vi "Robot_s Third Move.vi"(0 "Machine In":refnum<visa-resource-name>, 5 "Image Value From First Turn":dbl, 7 "Image  value From Second Turn":dbl, 9 "Index From First Move":i32, 11 "Index From Second Move":i32, 12 "error in":errorcluster) -> (4 "Machine Out":refnum<visa-resource-name>, 8 "Next Move":enum16{"Child's Turn", "Robot's Turn"}(ring), 15 "error out":errorcluster)   [LabVIEW 2018]
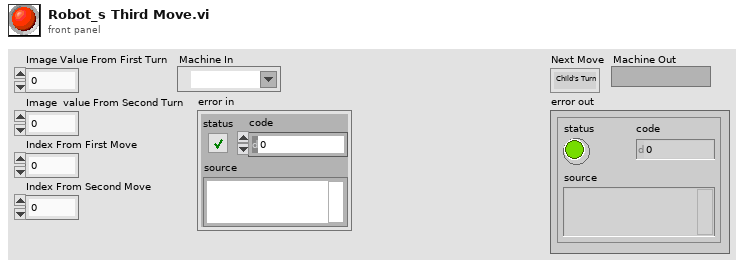
[diagram p1: front panel]
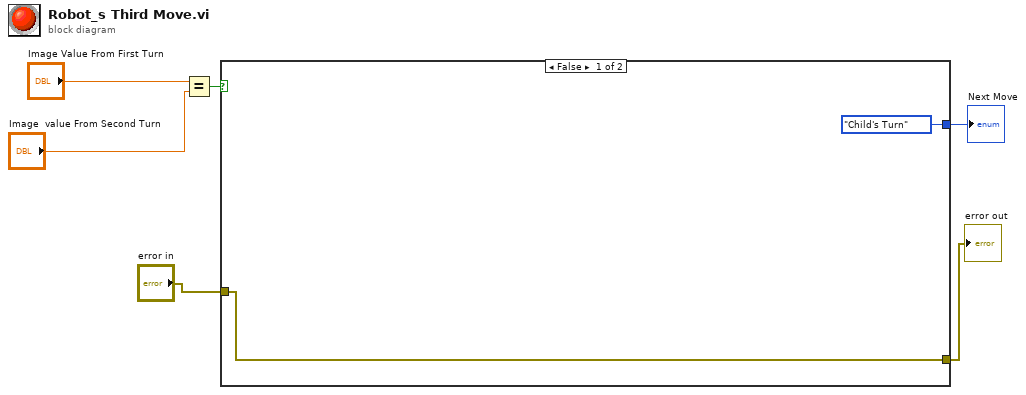
[diagram p0: block diagram]
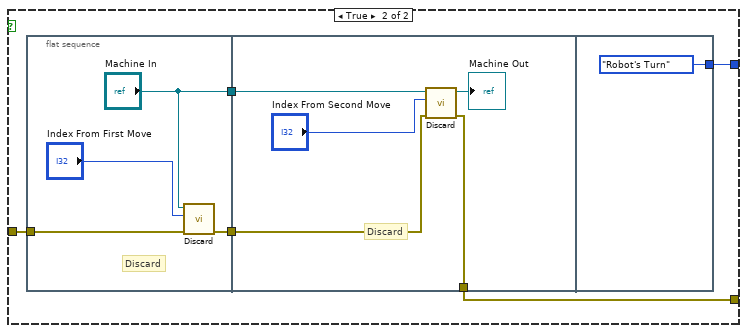
[diagram p2: hidden frame]
diagram:
  n1 = Equal?(x="Image Value From First Turn", y="Image  value From Second Turn") -> (x = y?=w6:bool)
  n2 = case shown="False" w6 {
    tunnel: [enum16{"Child's Turn", "Robot's Turn"}."Child's Turn" w13] -> w3
    tunnel: "error in" -> [w7 w10]
    tunnel: [w7 w9] -> w1
    frame False {
    }
    frame True {
      n3 = flat-sequence {
        tunnel: ["Machine In"] -> w12
        tunnel: [w15] -> w11
        tunnel: w10 -> [w14]
        tunnel: w12 -> [w22]
        tunnel: w11 -> [w20]
        tunnel: [w18] -> w9
        tunnel: [enum16{"Child's Turn", "Robot's Turn"}."Robot's Turn"] -> w13
        frame #0 {
          # "Discard"
          n4 = call "Discard.vi"("error in"=w14, "index"="Index From First Move", "Machine In"="Machine In") -> ("error out"=w15:errorcluster)  [unwired: 7 in, 1 out]
        }
        frame #1 {
          # "Discard"
          n5 = call "Discard.vi"("error in"=w20, "index"="Index From Second Move", "Machine In"=w22) -> ("error out"=w18:errorcluster, "Machine Out"=→"Machine Out":refnum<visa-resource-name>)  [unwired: 7 in]
        }
        frame #2 {
        }
      }
    }
  }
  "Next Move" <- w3
  "error out" <- w1
